vi "Fetch Single Measurement (Voltage).vi"(0 "VISA resource name":refnum<visa-resource-name>, 11 "error in (no error)":errorcluster) -> (4 "VISA resource name out":refnum<visa-resource-name>, 6 "DC Voltage":dbl, 8 "AC RMS Voltage":dbl, 10 "AC + DC RMS Voltage":dbl, 15 "error out":errorcluster)   [LabVIEW 2019, in "Agilent 681x Series.lvlib"]
doc: "Fetches and returns instantaneous voltage measurements.\n\n<B>Note:</B>\n\nUse this VI only with other low-level VIs. The high-level VIs automatically incorporate this functionality. This VI does not check the instrument status. If you want to check the instrument status, call the Error Query VI at the conclusion of the sequence."
uses:
  <instrlib>/Agilent 681x Series/Agilent 681x Series.lvlib
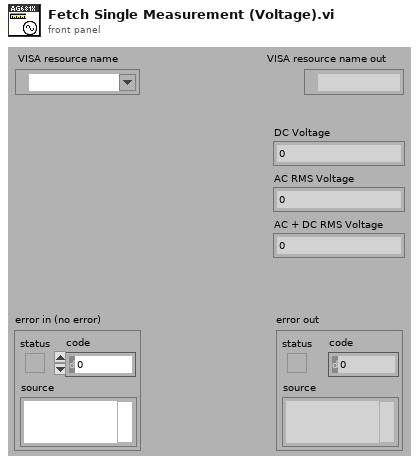
[diagram p1: front panel]
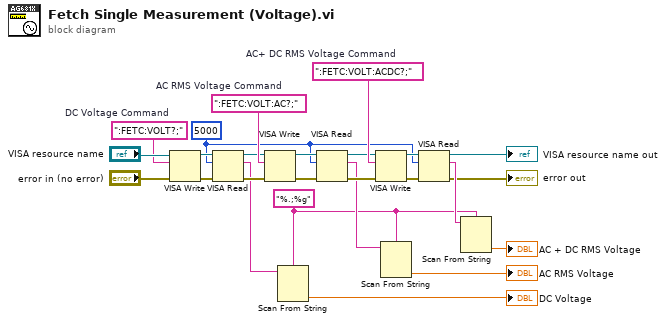
[diagram p0: block diagram]
diagram:
  w6 = "%.;%g"
  w14 = ":FETC:VOLT:ACDC?;"  # AC+ DC RMS Voltage Command
  w20 = ":FETC:VOLT:AC?;"  # AC RMS Voltage Command
  w11 = u32 5000 ("byte count")
  w21 = ":FETC:VOLT?;"  # DC Voltage Command
  n1 = VISA Write(VISA resource name="VISA resource name", write buffer=w21, error in (no error)="error in (no error)") -> (VISA resource name out=w22:refnum<visa-resource-name>, error out=w23:errorcluster)  [unwired: 1 out]
  n2 = VISA Read(VISA resource name=w22, byte count=w11, error in (no error)=w23) -> (VISA resource name out=w16:refnum<visa-resource-name>, read buffer=w9:string, error out=w15:errorcluster)  [unwired: 1 out]
  n3 = VISA Write(VISA resource name=w16, write buffer=w20, error in (no error)=w15) -> (VISA resource name out=w19:refnum<visa-resource-name>, error out=w10:errorcluster)  [unwired: 1 out]
  n4 = Scan From String(format string=w6, input string=w9) -> (output 1=→"DC Voltage":dbl)  [unwired: 3 in, 3 out]
  n5 = VISA Read(VISA resource name=w19, byte count=w11, error in (no error)=w10) -> (VISA resource name out=w12:refnum<visa-resource-name>, read buffer=w8:string, error out=w13:errorcluster)  [unwired: 1 out]
  n6 = VISA Write(VISA resource name=w12, write buffer=w14, error in (no error)=w13) -> (VISA resource name out=w17:refnum<visa-resource-name>, error out=w18:errorcluster)  [unwired: 1 out]
  n7 = Scan From String(format string=w6, input string=w8) -> (output 1=→"AC RMS Voltage":dbl)  [unwired: 3 in, 3 out]
  n8 = VISA Read(VISA resource name=w17, byte count=w11, error in (no error)=w18) -> (VISA resource name out=→"VISA resource name out":refnum<visa-resource-name>, read buffer=w7:string, error out=→"error out":errorcluster)  [unwired: 1 out]
  n9 = Scan From String(format string=w6, input string=w7) -> (output 1=→"AC + DC RMS Voltage":dbl)  [unwired: 3 in, 3 out]
